vi "carica bollettino.vi"(10 "output cluster":T1, 11 "Array":string[](array[string])) -> ()   [LabVIEW 2019]
uses:
  TypeDef/Control ref bollettino.ctl
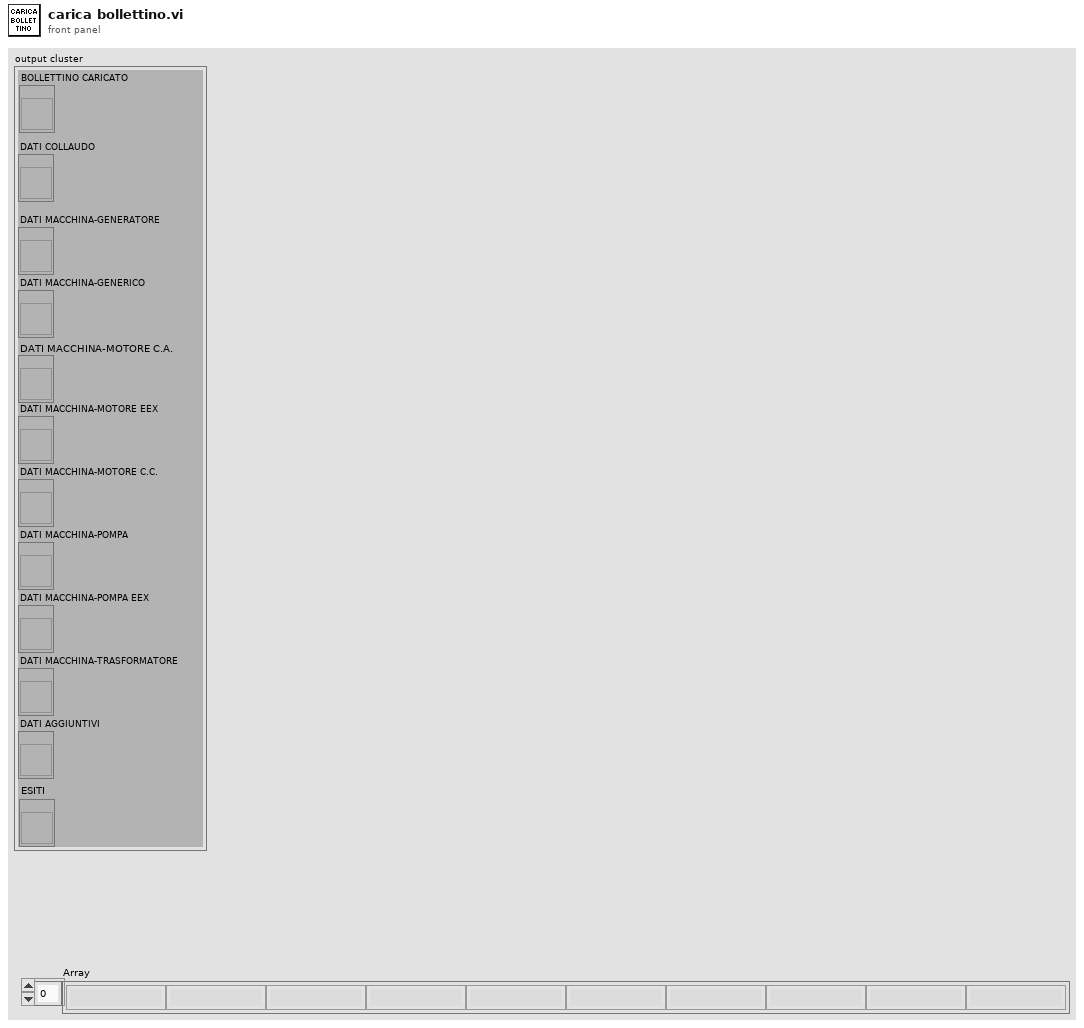
[diagram p1: front panel]
types:
  T1 = typedef "Control ref bollettino.ctl" = cluster{"BOLLETTINO CARICATO":refnum<vi>, "DATI COLLAUDO":refnum<vi>, "DATI MACCHINA-GENERATORE":refnum<vi>, "DATI MACCHINA-GENERICO":refnum<vi>, "DATI MACCHINA-MOTORE C.A.":refnum<vi>, "DATI MACCHINA-MOTORE EEX":refnum<vi>, "DATI MACCHINA-MOTORE C.C.":refnum<vi>, "DATI MACCHINA-POMPA":refnum<vi>, "DATI MACCHINA-POMPA EEX":refnum<vi>, "DATI MACCHINA-TRASFORMATORE":refnum<vi>, "DATI AGGIUNTIVI":refnum<vi>, "ESITI":refnum<vi>}
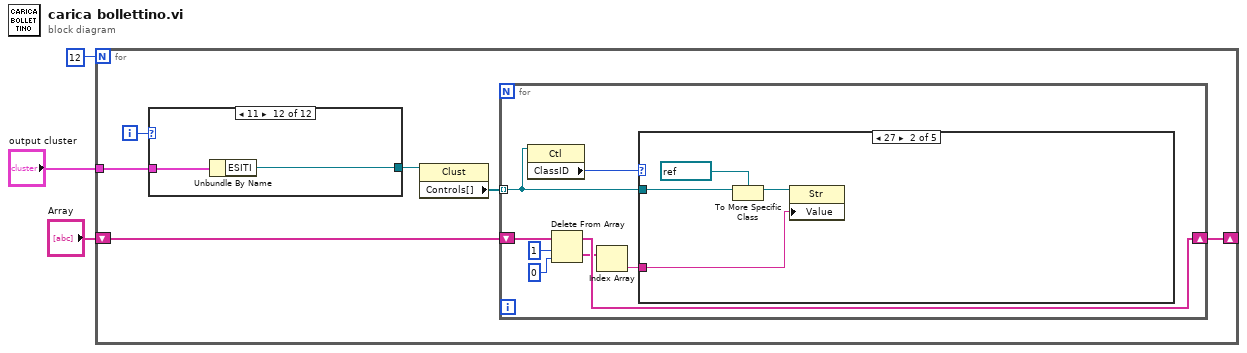
[diagram p0: block diagram]
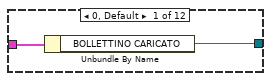
[diagram p2: hidden frame]
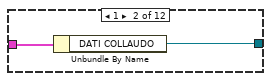
[diagram p3: hidden frame]
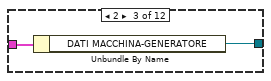
[diagram p4: hidden frame]
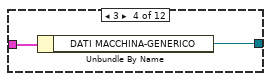
[diagram p5: hidden frame]
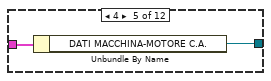
[diagram p6: hidden frame]
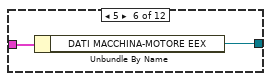
[diagram p7: hidden frame]
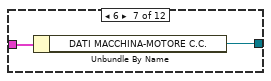
[diagram p8: hidden frame]
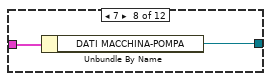
[diagram p9: hidden frame]
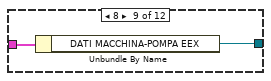
[diagram p10: hidden frame]
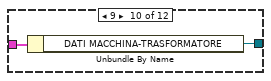
[diagram p11: hidden frame]
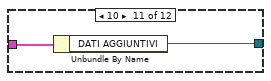
[diagram p12: hidden frame]
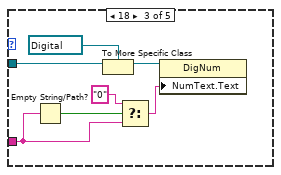
[diagram p14: hidden frame]
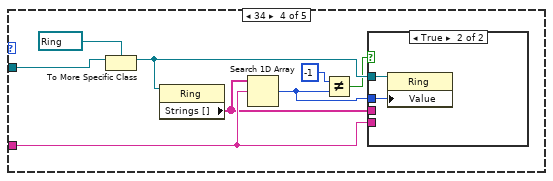
[diagram p15: hidden frame]
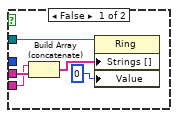
[diagram p16: hidden frame]
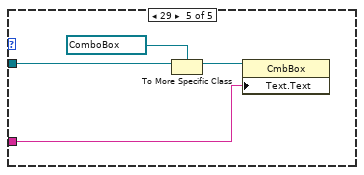
[diagram p17: hidden frame]
diagram:
  n1 = for {
    N: 12 -> [_]
    tunnel: "output cluster" -> [w5]
    shift-right: [w7] -> _
    shift-left: "Array" -> [w8]
    i -> [w6]
    n2 = case shown="11" w6 {
      tunnel: w5 -> [w11 w13 w15 w17 w19 w21 w23 w25 w27 w29 w31 w33]
      tunnel: [w10 w12 w14 w16 w18 w20 w22 w24 w26 w28 w30 w32] -> w4
      frame 0, Default {
        n3 = Unbundle By Name(w11) -> ("BOLLETTINO CARICATO"=w10:refnum<vi>)
      }
      frame 1 {
        n4 = Unbundle By Name(w13) -> ("DATI COLLAUDO"=w12:refnum<vi>)
      }
      frame 2 {
        n5 = Unbundle By Name(w15) -> ("DATI MACCHINA-GENERATORE"=w14:refnum<vi>)
      }
      frame 3 {
        n6 = Unbundle By Name(w17) -> ("DATI MACCHINA-GENERICO"=w16:refnum<vi>)
      }
      frame 4 {
        n7 = Unbundle By Name(w19) -> ("DATI MACCHINA-MOTORE C.A."=w18:refnum<vi>)
      }
      frame 5 {
        n8 = Unbundle By Name(w21) -> ("DATI MACCHINA-MOTORE EEX"=w20:refnum<vi>)
      }
      frame 6 {
        n9 = Unbundle By Name(w23) -> ("DATI MACCHINA-MOTORE C.C."=w22:refnum<vi>)
      }
      frame 7 {
        n10 = Unbundle By Name(w25) -> ("DATI MACCHINA-POMPA"=w24:refnum<vi>)
      }
      frame 8 {
        n11 = Unbundle By Name(w27) -> ("DATI MACCHINA-POMPA EEX"=w26:refnum<vi>)
      }
      frame 9 {
        n12 = Unbundle By Name(w29) -> ("DATI MACCHINA-TRASFORMATORE"=w28:refnum<vi>)
      }
      frame 10 {
        n13 = Unbundle By Name(w31) -> ("DATI AGGIUNTIVI"=w30:refnum<vi>)
      }
      frame 11 {
        n14 = Unbundle By Name(w33) -> ("ESITI"=w32:refnum<vi>)
      }
    }
    n15 = property class="Clust"(reference=w4) -> ("Controls[]"=w9:refnum<vi>[])  [unwired: 1 in, 2 out]
    n16 = for {
      tunnel: w9 -> [w40] mode=indexing
      shift-right: [w38] -> w7
      shift-left: w8 -> [w39]
      n17 = property class="Ctl"(reference=w40) -> ("ClassID"=w41:u32)  [unwired: 1 in, 2 out]
      n18 = Delete From Array(array=w39, length=1, index=0) -> (deleted portion=w37:string[], array with subset deleted=w38:string[])
      n19 = Index Array(array=w37) -> (element=w35:string)  [unwired: 1 in]
      n20 = case shown="27" w41 {
        tunnel: w40 -> [_ w44 w52 w59 w71]
        tunnel: w35 -> [_ w42 w48 w54 w68]
        frame 0, Default {
        }
        frame 27 {
          n21 = To More Specific Class(target class=refnum<vi> refnum ("String"), reference=w44) -> (specific class reference=w43:refnum<vi>)  [unwired: 1 in, 1 out]
          n22 = property class="Str"(reference=w43, "Value"=w42) -> ()  [unwired: 1 in, 2 out]
        }
        frame 18 {
          n23 = Empty String/Path?(string/path=w48) -> (empty?=w49:bool)
          n24 = To More Specific Class(target class=refnum<vi> refnum ("Numeric Control"), reference=w52) -> (specific class reference=w50:refnum<vi>)  [unwired: 1 in, 1 out]
          n25 = Select(t="0", s=w49, f=w48) -> (s? t:f=w46:string)
          n26 = property class="DigNum"(reference=w50, "NumText.Text"=w46) -> ()  [unwired: 1 in, 2 out]
        }
        frame 34 {
          n27 = To More Specific Class(target class=refnum<vi> refnum ("Menu Ring"), reference=w59) -> (specific class reference=w58:refnum<vi>)  [unwired: 1 in, 1 out]
          n28 = property class="Ring"(reference=w58) -> ("Strings []"=w53:string[])  [unwired: 1 in, 2 out]
          n29 = Search 1D Array(1D array=w53, element=w54) -> (index of element=w56:i32)  [unwired: 1 in]
          n30 = Not Equal?(x=-1, y=w56) -> (x != y?=w57:bool)
          n31 = case shown="True" w57 {
            tunnel: w58 -> [w65 w67]
            tunnel: w56 -> [_ w66]
            tunnel: w54 -> [w63 _]
            tunnel: w53 -> [w64 _]
            frame False {
              n32 = Build Array (concatenate)(w63, w64) -> (w62:string[])
              n33 = property class="Ring"(reference=w65, "Strings []"=w62, "Value"=0) -> ()  [unwired: 1 in, 2 out]
            }
            frame True {
              n34 = property class="Ring"(reference=w67, "Value"=w66) -> ()  [unwired: 1 in, 2 out]
            }
          }
        }
        frame 29 {
          n35 = To More Specific Class(target class=refnum<vi> refnum ("FILE TARATURA"), reference=w71) -> (specific class reference=w70:refnum<vi>)  [unwired: 1 in, 1 out]
          n36 = property class="CmbBox"(reference=w70, "Text.Text"=w68) -> ()  [unwired: 1 in, 2 out]
        }
      }
    }
  }
